vi "Get Signal Names from DVR.vi"(8 "error in (no error)":errorcluster, 11 "Data Value Reference in":T1) -> (0 "error out":errorcluster, 2 "Signal List":string[](array[string]), 3 "Data Value Reference out":T1)   [LabVIEW 2011]
uses:
  Controls/DVR of CSV Tests Data.ctl
  Controls/CSVs Tests Data.ctl
  Controls/Test Column Data.ctl
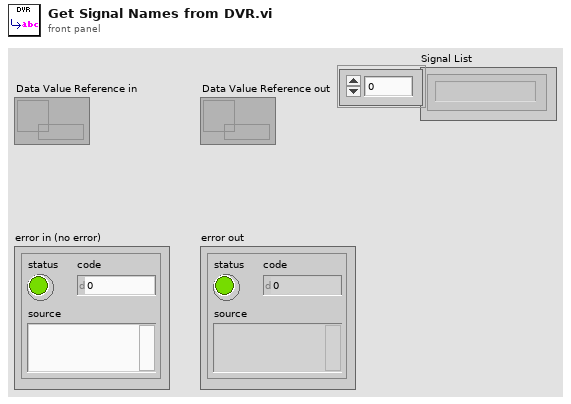
[diagram p1: front panel]
types:
  T1 = typedef "DVR of CSV Tests Data.ctl" = refnum<data-value>
  T2 = typedef "CSVs Tests Data.ctl" = cluster{"Test Data":T3[], "CsvPath":path, "LogPath":path, "Pass?":bool, "Error":errorcluster}
  T3 = typedef "Test Column Data.ctl" = cluster{"Chn":string, "ExpVals":dbl[], "TimeStamps":i64[], "NegTol":dbl, "PosTol":dbl}
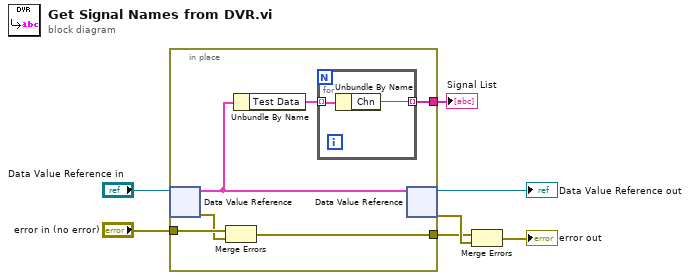
[diagram p0: block diagram]
diagram:
  n1 = in-place {
    in-place-border: "error in (no error)" -> [w13]
    in-place-border: [w10] -> w4
    in-place-border: [w8] -> w1
    n2 = in-place-dvr #1("Data Value Reference in") -> (w11:T2, w12:errorcluster)
    n3 = Merge Errors(w13, w12) -> (w10:errorcluster)
    n4 = Unbundle By Name(w11) -> ("Test Data"=w9:T3[])
    n5 = for {
      tunnel: w9 -> [w15] mode=indexing
      tunnel: [w14] -> w8 mode=indexing
      n6 = Unbundle By Name(w15) -> ("Chn"=w14:string)
    }
    n7 = in-place-dvr #1(w11) -> (→"Data Value Reference out":T1, w5:errorcluster)
  }
  "Signal List" <- w1
  n8 = Merge Errors(w4, w5) -> (→"error out":errorcluster)
